vi "Get Interval Duration.vi"(5 "Interval":T1={"Interval Type"=enum."Walk", "Duration"=20.0, " Mode"=enum."Stim", "Alt Period"=0.0}) -> (1 "Interval Duration (ms)":dbl[unit], 2 "Interval Duration (s)":dbl[unit])   [LabVIEW 2019]
uses:
  Controls/Protocol Interval.ctl
  Controls/Stim Interval Mode.ctl
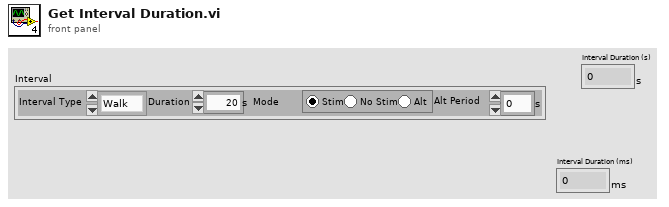
[diagram p1: front panel]
types:
  T1 = typedef "Protocol Interval.ctl" = cluster{"Interval Type":enum16{"Walk", "Rest"}, "Duration":dbl[unit], " Mode":T2, "Alt Period":dbl[unit]}
  T2 = typedef "Stim Interval Mode.ctl" = enum32{"Stim", "No Stim", "Alternating"}
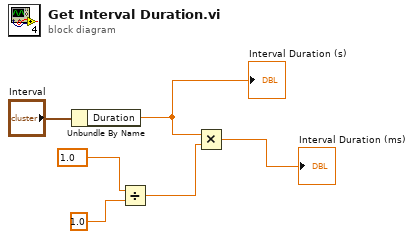
[diagram p0: block diagram]
diagram:
  n1 = Unbundle By Name("Interval") -> ("Duration"=w6:dbl[unit])
  "Interval Duration (s)" <- w6
  n2 = Divide(x=dbl[unit] 1.0 ("y"), y=dbl[unit] 1.0) -> (x/y=w2:dbl)
  n3 = Multiply(x=w6, y=w2) -> (x*y=→"Interval Duration (ms)":dbl[unit])
